vi "LDO Trigger Events.vi"(0 "All Data":T1 {"PLC Data"."PLC Data - LDO"."Timing"."Absolute Time" format="%<%H:%M:%S%3u>t"; "PLC Data"."PLC Data - LDO"."Timing"."Display Time" format="%#.20f"; "PLC Data"."PLC Data - LDO"."Timing"."Test Time Ref" format="%#.20f"; "PLC Data"."PLC Data - LDO"."Timing"."Precondition Time Ref" format="%#.20f"; "PLC Data"."PLC Data - LDO"."Timing"."First Call Time Ref" format="%#.20f"; "PLC Data"."PLC Data - FVIR"."Timing"."Absolute Time" format="%<%H:%M:%S%3u>t"; "PLC Data"."PLC Data - FVIR"."Timing"."Display Time" format="%#.20f"; "PLC Data"."PLC Data - FVIR"."Timing"."Test Time Ref" format="%#.20f"; "PLC Data"."PLC Data - FVIR"."Timing"."Precondition Time Ref" format="%#.20f"; "PLC Data"."PLC Data - FVIR"."Timing"."First Call Time Ref" format="%#.20f"}, 2 "Event Booleans in":T16, 7 "error in":errorcluster, 9 "Rotary Actuator (ON/OFF)":refnum<vi>, 11 "Start recording data":refnum<vi>, 13 "Burner ON Ref":refnum<vi>, 14 "Burner ON":bool, 15 "0.8 ML Ref":refnum<vi>, 17 "1.1 ML Ref":refnum<vi>, 19 "1.33 ML Ref":refnum<vi>) -> (20 "All Data Output":T1 {"PLC Data"."PLC Data - LDO"."Timing"."Absolute Time" format="%<%H:%M:%S%3u>t"; "PLC Data"."PLC Data - LDO"."Timing"."Display Time" format="%#.20f"; "PLC Data"."PLC Data - LDO"."Timing"."Test Time Ref" format="%#.20f"; "PLC Data"."PLC Data - LDO"."Timing"."Precondition Time Ref" format="%#.20f"; "PLC Data"."PLC Data - LDO"."Timing"."First Call Time Ref" format="%#.20f"; "PLC Data"."PLC Data - FVIR"."Timing"."Absolute Time" format="%<%H:%M:%S%3u>t"; "PLC Data"."PLC Data - FVIR"."Timing"."Display Time" format="%#.20f"; "PLC Data"."PLC Data - FVIR"."Timing"."Test Time Ref" format="%#.20f"; "PLC Data"."PLC Data - FVIR"."Timing"."Precondition Time Ref" format="%#.20f"; "PLC Data"."PLC Data - FVIR"."Timing"."First Call Time Ref" format="%#.20f"}, 22 "Event Booleans out":T16, 27 "error out":errorcluster)   [LabVIEW 2020]
uses:
  Event Booleans.ctl
  Modbus/Modbus All Data.ctl
  Modbus/Modbus PLC Data All.ctl
  Modbus/Modbus FVIR Control.ctl
  Modbus/Modbus Timing.ctl
  <vilib>/Utility/miscctls.llb/LVDateTimeRec.ctl
  Modbus/Modbus LDO Control.ctl
  WritingDataFile/Data to Save.ctl
  Terminate Conditions Cluster.ctl
  Drivers/Inficon Transmitter/Type Definitions/Inficon Data.ctl
  Modbus/Modbus Gas Meter Data.ctl
  Drivers/Alicat LabVIEW Drivers 2v1/Sub-VIs/Data Cluster.ctl
  Drivers/Alicat LabVIEW Drivers 2v1/Sub-VIs/Units of Measure.ctl
  Gas_Rate/HEWH ANSI Rate.ctl
  Drivers/Resideo Gas Valve/Type Definitions/Vesta Info.ctl
  Agilent Data.ctl
panel:
  # "Totalizer Timer"
  # "Totalizer Timer"
  # "Natural Gas"
  # "Propane"
  # "Totalizer Timer"
  # "Totalizer Timer"
  # "Natural Gas"
  # "Propane"
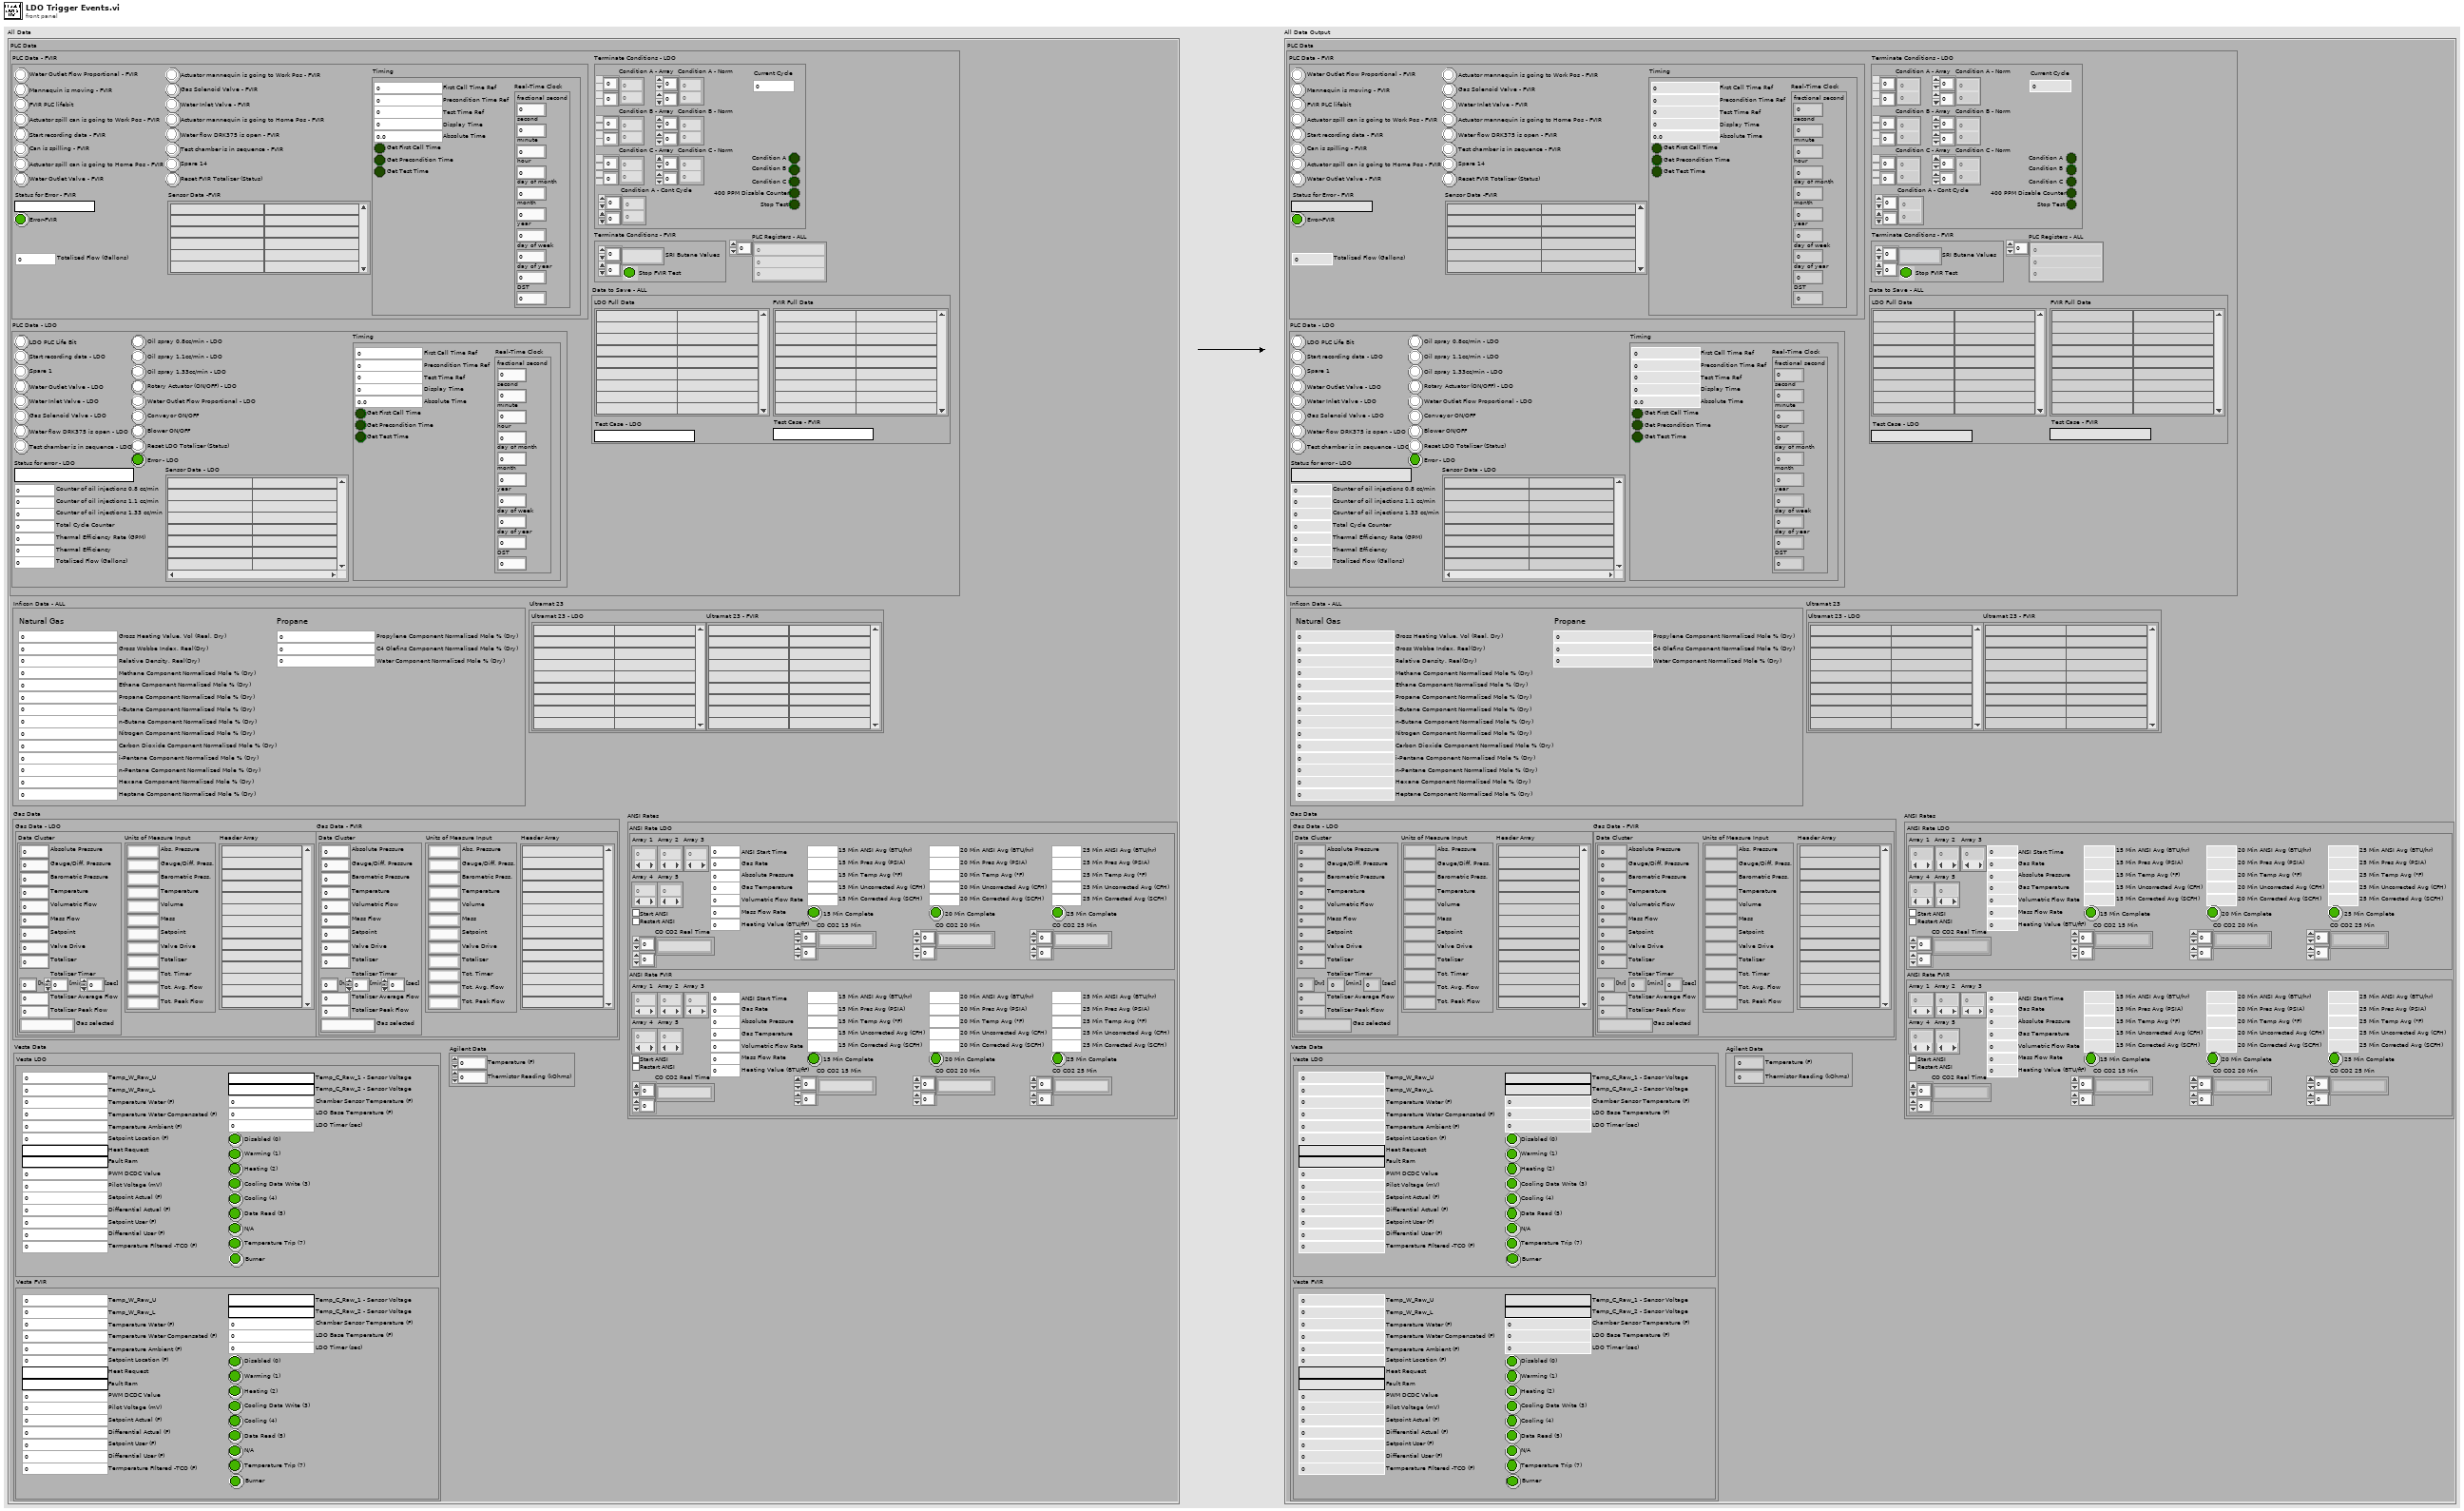
[diagram p1: front panel]
types:
  T1 = typedef "Modbus All Data.ctl" = cluster{"PLC Data":T2, "Inficon Data - ALL":T9, "Gas Data":cluster{"Gas Data - LDO":T10, "Gas Data - FVIR":T10}, "Ultramat 23":cluster{"Ultramat 23 - LDO":string[][], "Ultramat 23 - FVIR":string[][]}, "ANSI Rates":cluster{"ANSI Rate LDO":T13, "ANSI Rate FVIR":T13}, "Vesta Data":cluster{"Vesta LDO":T14, "Vesta FVIR":T14}, "Agilent Data":T15}
  T2 = typedef "Modbus PLC Data All.ctl" = cluster{"PLC Data - FVIR":T3, "PLC Data - LDO":T6, "PLC Registers - ALL":i16[], "Data to Save - ALL":T7, "Terminate Conditions - LDO":T8, "Terminate Conditions - FVIR":cluster{"SRI Butane Values":string[][], "Stop FVIR Test":bool}}
  T3 = typedef "Modbus FVIR Control.ctl" = cluster{"Reset FVIR Totalizer (Status)":bool, "Spare 14":bool, "Actuator mannequin is going to Work Pos - FVIR":bool, "Actuator mannequin is going to Home Pos - FVIR":bool, "Test chamber is in sequence - FVIR ":bool, "Water flow DRK375 is open - FVIR":bool, "Gas Solenoid Valve - FVIR":bool, "Water Inlet Valve - FVIR":bool, "Water Outlet Flow Proportional - FVIR":bool, "Start recording data - FVIR":bool, "Actuator spill can is going to Work Pos - FVIR":bool, "Actuator spill can is going to Home Pos - FVIR":bool, "Water Outlet Valve - FVIR":bool, "Can is spilling - FVIR":bool, "Mannequin is moving - FVIR":bool, "FVIR PLC lifebit":bool, "Status for Error - FVIR":string, "Error-FVIR":bool, "Sensor Data -FVIR":string[][], "Totalized Flow (Gallons)":dbl, "Timing":T4}
  T4 = typedef "Modbus Timing.ctl" = cluster{"First Call Time Ref":dbl, "Precondition Time Ref":dbl, "Test Time Ref":dbl, "Get First Call Time":bool, "Get Precondition Time":bool, "Get Test Time":bool, "Display Time":dbl, "Real-Time Clock":T5, "Absolute Time":dbl}
  T5 = typedef "LVDateTimeRec.ctl" = cluster{"fractional second":dbl, "second":i32, "minute":i32, "hour":i32, "day of month":i32, "month":i32, "year":i32, "day of week":i32, "day of year":i32, "DST":i32}
  T6 = typedef "Modbus LDO Control.ctl" = cluster{"LDO PLC Life Bit":bool, "Start recording data - LDO":bool, "Spare 1":bool, "Water Outlet Valve - LDO":bool, "Water Inlet Valve - LDO":bool, "Gas Solenoid Valve - LDO":bool, "Water flow DRK375 is open - LDO":bool, "Test chamber is in sequence - LDO":bool, "Oil spray 0.8cc/min - LDO":bool, "Oil spray 1.1cc/min - LDO":bool, "Oil spray 1.33cc/min - LDO":bool, "Rotary Actuator (ON/OFF) - LDO":bool, "Water Outlet Flow Proportional - LDO":bool, "Conveyor ON/OFF":bool, "Blower ON/OFF":bool, "Reset LDO Totalizer (Status)":bool, "Status for error - LDO":string, "Error - LDO":bool, "Sensor Data - LDO":string[][], "Thermal Efficiency Rate (GPM)":dbl, "Thermal Efficiency":dbl, "Totalized Flow (Gallons)":dbl, "Counter of oil injections 1.33 cc/min":u16, "Total Cycle Counter":u16, "Counter of oil injections 1.1 cc/min":u16, "Counter of oil injections 0.8 cc/min":u16, "Timing":T4}
  T7 = typedef "Data to Save.ctl" = cluster{"LDO Full Data":string[][], "FVIR Full Data":string[][], "Test Case - FVIR":string, "Test Case - LDO":string}
  T8 = typedef "Terminate Conditions Cluster.ctl" = cluster{"Condition B - Array":dbl[][], "Current Cycle":u16, "Condition C - Array":dbl[][], "Condition A - Array":dbl[][], "400 PPM Disable Counter":bool, "Condition A - Norm":dbl[][], "Condition B - Norm":dbl[][], "Condition C - Norm":dbl[][], "Condition A":bool, "Condition B":bool, "Condition C":bool, "Condition A - Cont Cycle":dbl[][], "Stop Test":bool}
  T9 = typedef "Inficon Data.ctl" = cluster{"Gross Heating Value, Vol (Real, Dry)":dbl, "Nitrogen Component Normalized Mole % (Dry)":dbl, "Methane Component Normalized Mole % (Dry)":dbl, "Carbon Dioxide Component Normalized Mole % (Dry)":dbl, "Ethane Component Normalized Mole % (Dry)":dbl, "Propane Component Normalized Mole % (Dry)":dbl, "i-Pentane Component Normalized Mole % (Dry)":dbl, "i-Butane Component Normalized Mole % (Dry)":dbl, "n-Butane Component Normalized Mole % (Dry)":dbl, "n-Pentane Component Normalized Mole % (Dry)":dbl, "Hexane Component Normalized Mole % (Dry)":dbl, "Heptane Component Normalized Mole % (Dry)":dbl, "Gross Wobbe Index, Real(Dry)":dbl, "Relative Density, Real(Dry)":dbl, "Propylene Component Normalized Mole % (Dry)":dbl, "C4 Olefins Component Normalized Mole % (Dry)":dbl, "Water Component Normalized Mole % (Dry)":dbl}
  T10 = typedef "Modbus Gas Meter Data.ctl" = cluster{"Data Cluster":T11, "Units of Measure Input":T12, "Header Array":string[]}
  T11 = typedef "Data Cluster.ctl" = cluster{"Absolute Pressure":dbl, "Gauge/Diff. Pressure":dbl, "Barometric Pressure":dbl, "Temperature":dbl, "Volumetric Flow":dbl, "Mass Flow":dbl, "Setpoint":dbl, "Valve Drive":dbl, "Totalizer":dbl, "[hr]":dbl, "[min]":dbl, "[sec]":dbl, "Totalizer Average Flow":dbl, "Totalizer Peak Flow":dbl, "Gas selected":string}
  T12 = typedef "Units of Measure.ctl" = cluster{"Abs. Pressure":string, "Gauge/Diff. Press.":string, "Barometric Press.":string, "Temperature":string, "Volume":string, "Mass":string, "Setpoint":string, "Valve Drive":string, "Totalizer":string, "Tot. Timer":string, "Tot. Avg. Flow":string, "Tot. Peak Flow":string}
  T13 = typedef "HEWH ANSI Rate.ctl" = cluster{"Array 1":dbl[], "Array 3":dbl[], "Array 2":dbl[], "Start ANSI":bool, "ANSI Start Time":dbl, "Restart ANSI":bool, "15 Min ANSI Avg (BTU/hr)":dbl, "20 Min ANSI Avg (BTU/hr)":dbl, "25 Min ANSI Avg (BTU/hr)":dbl, "Absolute Pressure":dbl, "Gas Temperature":dbl, "Volumetric Flow Rate":dbl, "Mass Flow Rate":dbl, "Array 4":dbl[], "Array 5":dbl[], "Gas Rate":dbl, "15 Min Pres Avg (PSIA)":dbl, "20 Min Pres Avg (PSIA)":dbl, "25 Min Pres Avg (PSIA)":dbl, "15 Min Temp Avg (°F) ":dbl, "20 Min Temp Avg (°F)":dbl, "25 Min Temp Avg (°F)":dbl, "15 Min Uncorrected Avg (CFH)":dbl, "20 Min Uncorrected Avg (CFH)":dbl, "25 Min Uncorrected Avg (CFH)":dbl, "15 Min Corrected Avg (SCFH)":dbl, "20 Min Corrected Avg (SCFH)":dbl, "25 Min Corrected Avg (SCFH)":dbl, "15 Min Complete":bool, "20 Min Complete":bool, "25 Min Complete":bool, "Heating Value (BTU/ft³)":dbl, "CO CO2 15 Min":string[][], "CO CO2 20 Min":string[][], "CO CO2 25 Min":string[][], "CO CO2 Real Time":string[][]}
  T14 = typedef "Vesta Info.ctl" = cluster{"Temp_W_Raw_U":u16, "Temp_W_Raw_L":u16, "Temperature Water (F)":dbl, "Temperature Water Compensated (F)":dbl, "Temperature Ambient (F)":dbl, "Setpoint Location (F)":dbl, "Heat Request":string, "Fault Ram":string, "PWM DCDC Value":u16, "Pilot Voltage (mV)":dbl, "Setpoint Actual (F)":dbl, "Differential Actual (F)":dbl, "Setpoint User (F)":dbl, "Differential User (F)":dbl, "Termperature FIltered -TCO (F)":dbl, "Temp_C_Raw_1 - Sensor Voltage":string, "Temp_C_Raw_2 - Sensor Voltage":string, "Chamber Sensor Temperature (F)":dbl, "LDO Base Temperature (F)":dbl, "LDO Timer (sec)":i16, "Disabled (0)":bool, "Warming (1)":bool, "Heating (2)":bool, "Cooling Data Write (3)":bool, "Cooling (4)":bool, "Data Read (5)":bool, "N/A":bool, "Temperature Trip (7)":bool, "Burner":bool}
  T15 = typedef "Agilent Data.ctl" = cluster{"Temperature (F)":dbl, "Thermistor Reading (kOhms)":dbl}
  T16 = typedef "Event Booleans.ctl" = cluster{"Burner ON - LDO":bool, "0.8 ml Bool":bool, "1.1 Bool":bool, "1.33 Bool":bool, "Start recording data-LDO":bool, "Rotary Actuator (ON/OFF)":bool, "Burner ON - FVIR":bool, "Start recording data -FVIR ":bool}
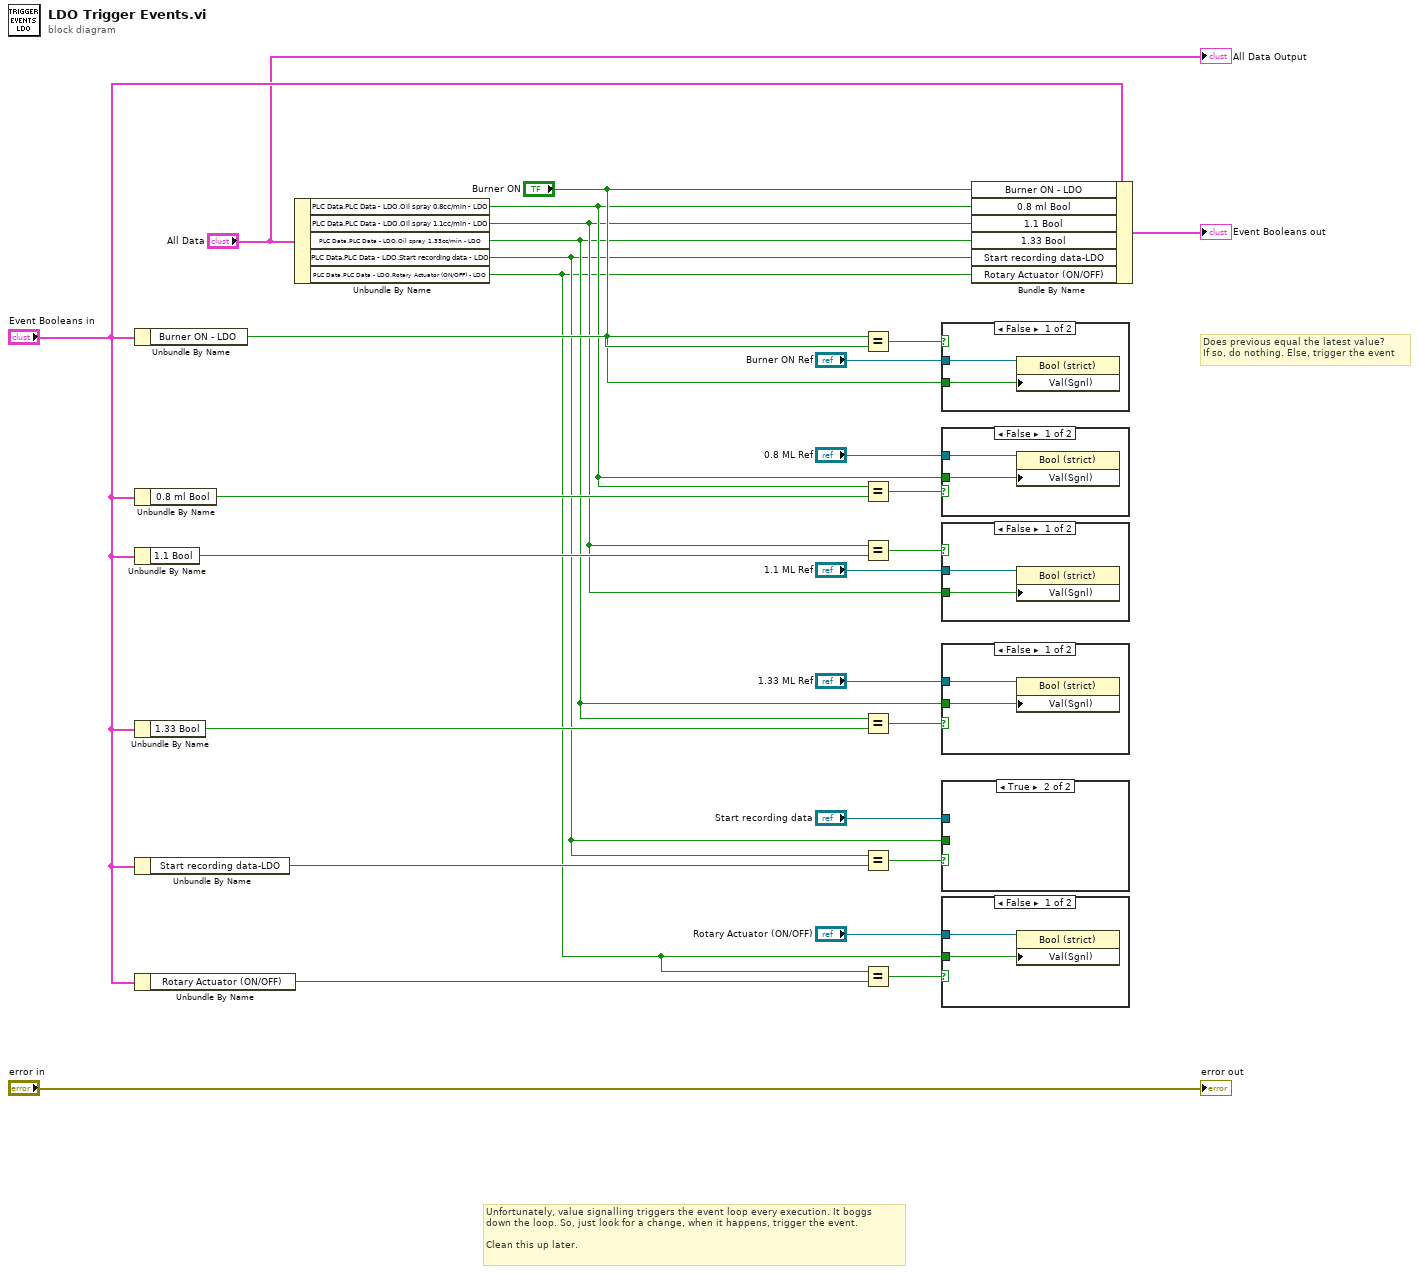
[diagram p0: block diagram]
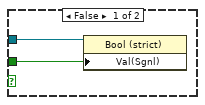
[diagram p3: hidden frame]
diagram:
  # "Does previous equal the latest value?\nIf so, do nothing. Else, trigger the event"
  # "Unfortunately, value signalling triggers the event loop every execution. It boggs\ndown the loop. So, just look for a change, when it happens, trigger the event. \n\nClean this up later."
  n1 = Unbundle By Name("Event Booleans in") -> ("Burner ON - LDO"=w19:bool)
  n2 = Unbundle By Name("Event Booleans in") -> ("0.8 ml Bool"=w18:bool)
  n3 = Unbundle By Name("Event Booleans in") -> ("1.1 Bool"=w17:bool)
  n4 = Unbundle By Name("Event Booleans in") -> ("1.33 Bool"=w16:bool)
  n5 = Unbundle By Name("Event Booleans in") -> ("Start recording data-LDO"=w11:bool)
  n6 = Unbundle By Name("Event Booleans in") -> ("Rotary Actuator (ON/OFF)"=w7:bool)
  n7 = Unbundle By Name("All Data") -> ("PLC Data.PLC Data - LDO.Oil spray 0.8cc/min - LDO"=w6:bool, "PLC Data.PLC Data - LDO.Oil spray 1.1cc/min - LDO"=w5:bool, "PLC Data.PLC Data - LDO.Oil spray 1.33cc/min - LDO"=w4:bool, "PLC Data.PLC Data - LDO.Start recording data - LDO"=w3:bool, "PLC Data.PLC Data - LDO.Rotary Actuator (ON/OFF) - LDO"=w2:bool)
  n8 = Equal?(x="Burner ON", y=w19) -> (x = y?=w24:bool)
  n9 = Equal?(x=w6, y=w18) -> (x = y?=w26:bool)
  n10 = Equal?(x=w5, y=w17) -> (x = y?=w28:bool)
  n11 = Equal?(x=w4, y=w16) -> (x = y?=w27:bool)
  n12 = Equal?(x=w3, y=w11) -> (x = y?=w13:bool)
  n13 = Equal?(x=w2, y=w7) -> (x = y?=w8:bool)
  n14 = case shown="False" w24 {
    tunnel: "Burner ON" -> [w30 _]
    tunnel: "Burner ON Ref" -> [w29 _]
    frame False {
      n15 = property on="Property Node" class="Bool (strict)"(reference=w29, "Val(Sgnl)"=w30) -> ()  [unwired: 1 in, 2 out]
    }
    frame True {
    }
  }
  n16 = case shown="False" w26 {
    tunnel: w6 -> [w32 _]
    tunnel: "0.8 ML Ref" -> [w31 _]
    frame False {
      n17 = property on="Property Node" class="Bool (strict)"(reference=w31, "Val(Sgnl)"=w32) -> ()  [unwired: 1 in, 2 out]
    }
    frame True {
    }
  }
  n18 = case shown="False" w28 {
    tunnel: w5 -> [w34 _]
    tunnel: "1.1 ML Ref" -> [w33 _]
    frame False {
      n19 = property on="Property Node" class="Bool (strict)"(reference=w33, "Val(Sgnl)"=w34) -> ()  [unwired: 1 in, 2 out]
    }
    frame True {
    }
  }
  n20 = case shown="False" w27 {
    tunnel: w4 -> [w36 _]
    tunnel: "1.33 ML Ref" -> [w35 _]
    frame False {
      n21 = property on="Property Node" class="Bool (strict)"(reference=w35, "Val(Sgnl)"=w36) -> ()  [unwired: 1 in, 2 out]
    }
    frame True {
    }
  }
  n22 = case shown="True" w13 {
    tunnel: w3 -> [w37 _]
    tunnel: "Start recording data" -> [w38 _]
    frame False {
      n23 = property on="Property Node" class="Bool (strict)"(reference=w38, "Val(Sgnl)"=w37) -> ()  [unwired: 1 in, 2 out]
    }
    frame True {
    }
  }
  n24 = case shown="False" w8 {
    tunnel: w2 -> [w39 _]
    tunnel: "Rotary Actuator (ON/OFF)" -> [w40 _]
    frame False {
      n25 = property on="Property Node" class="Bool (strict)"(reference=w40, "Val(Sgnl)"=w39) -> ()  [unwired: 1 in, 2 out]
    }
    frame True {
    }
  }
  n26 = Bundle By Name(cluster="Event Booleans in", "Burner ON - LDO"="Burner ON", "0.8 ml Bool"=w6, "1.1 Bool"=w5, "1.33 Bool"=w4, "Start recording data-LDO"=w3, "Rotary Actuator (ON/OFF)"=w2) -> (→"Event Booleans out":T16)
  "error out" <- "error in"
  "All Data Output" <- "All Data"
